vi "line_spectrum.vi"(1 "Image":dbl[][](graph)=array476x2048[974848 elements]) -> (0 "Mean intensity per pixel":cluster{"Ramp Pattern":dbl[], dbl[]}[](graph)=[{"Ramp Pattern"=array[2048 elements], array[2048 elements]}, {"Ramp Pattern"=[767.5, 767.5], [0.0, 100.0]}, {"Ramp Pattern"=[932.5, 932.5], [0.0, 100.0]}, {"Ramp Pattern"=[850.0, 850.0], [0.0, 100.0]}])   [LabVIEW 2017]
uses:
  <vilib>/Analysis/1siggen.llb/Ramp Pattern by Samples.vi
  <vilib>/Analysis/baseanly.llb/Mean (DBL).vi
  <vilib>/Analysis/NI_AALBase.lvlib
panel:
  out "MaxPI (%)":dbl=87.1199407497374 format="%0.1f"
  in  "Source Bandwidth (nm)":i32=165
  in  "Source Center wavelength (nm)":i32=850
  in  "Spec. Bandwidth (nm)":i32=180
  in  "Spec. Center wavelength (nm)":i32=840
  out "MPI (%)":dbl=43.9106688028624 format="%0.1f"
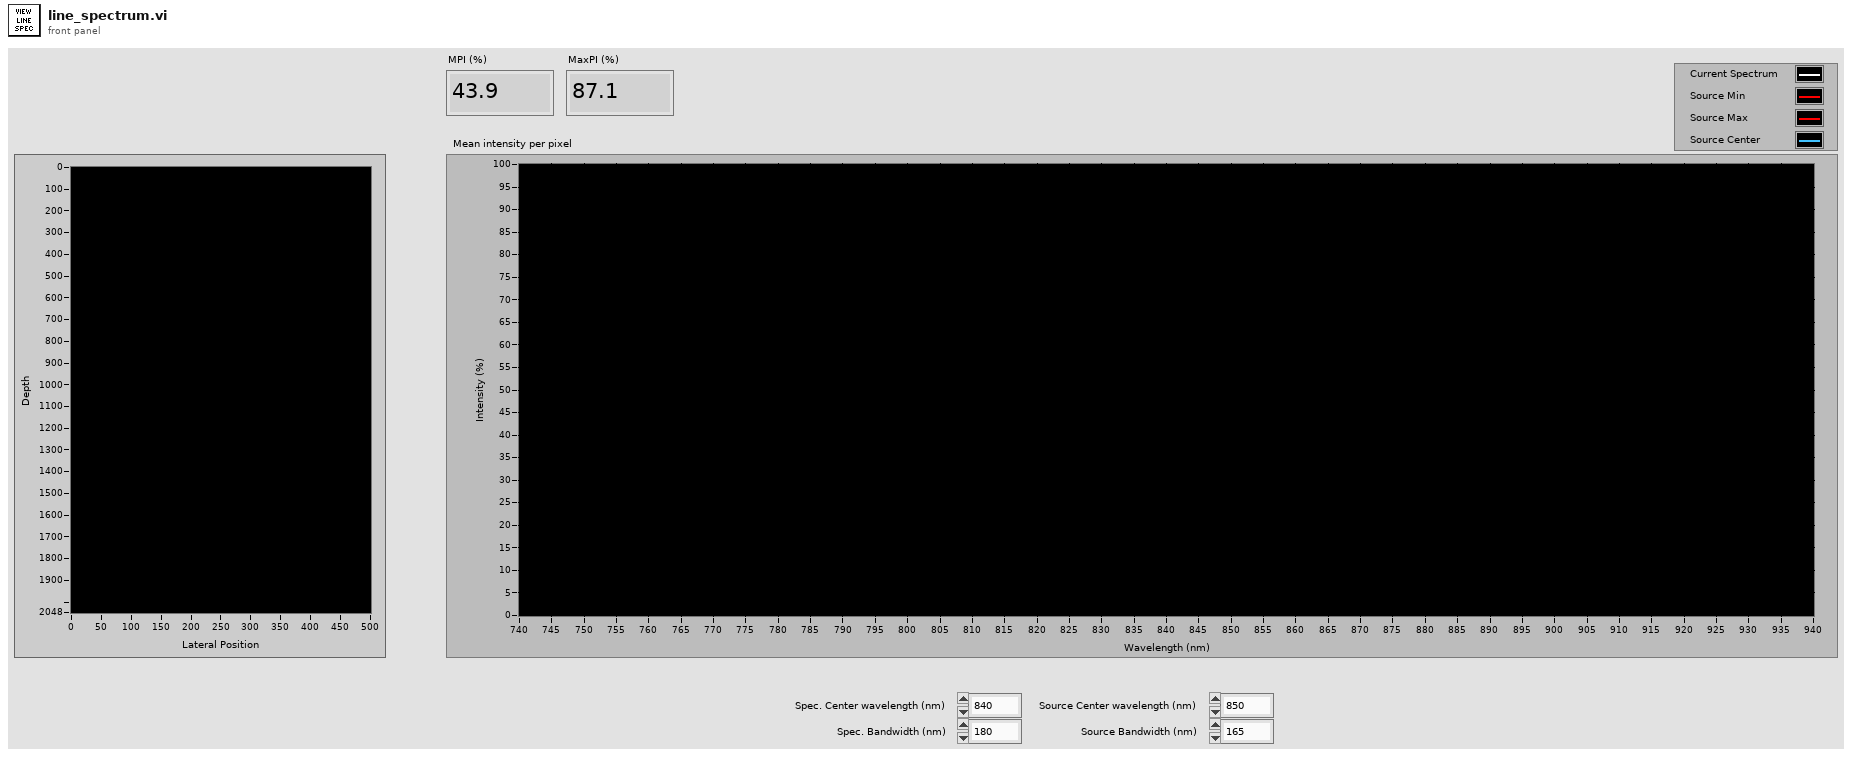
[diagram p1: front panel]
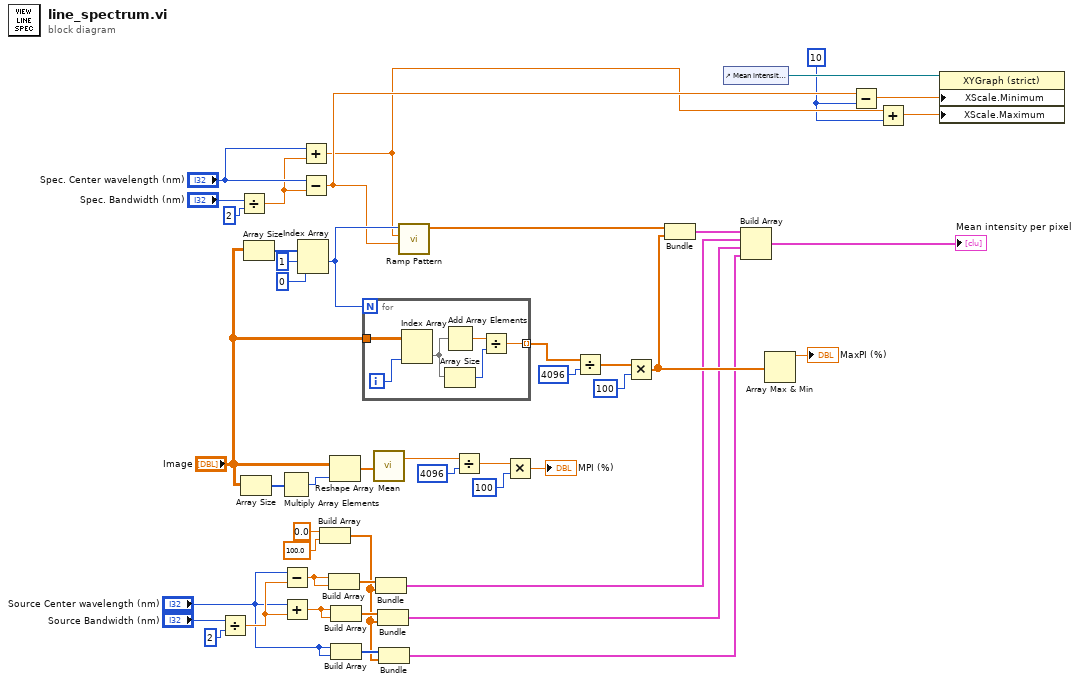
[diagram p0: block diagram]
diagram:
  w1 = 10
  n1 = Divide(x="Source Bandwidth (nm)", y=2) -> (x/y=w24:dbl)
  n2 = Divide(x="Spec. Bandwidth (nm)", y=2) -> (x/y=w26:dbl)
  n3 = Array Size(array="Image") -> (size(s)=w46:i32[])
  n4 = Array Size(array="Image") -> (size(s)=w43:i32[])
  n5 = Multiply Array Elements(1:w46) -> (0:w45:i32)
  n6 = Subtract(x="Source Center wavelength (nm)", y=w24) -> (x-y=w20:dbl)
  n7 = Add(x="Source Center wavelength (nm)", y=w24) -> (x+y=w17:dbl)
  n8 = Index Array(array=w43, index #1=1 ("index"), index #2=0 ("index")) -> (element #1=w39:i32)  [unwired: 1 out]
  n9 = Add(x="Spec. Center wavelength (nm)", y=w26) -> (x+y=w2:dbl)
  n10 = Subtract(x="Spec. Center wavelength (nm)", y=w26) -> (x-y=w3:dbl)
  n11 = Build Array(0.0 ("element"), 100.0 ("element")) -> (w10:dbl[])
  n12 = Build Array(w20, w20) -> (w16:dbl[])
  n13 = Reshape Array("Image", w45) -> (w8:dbl[])
  n14 = Build Array(w17, w17) -> (w15:dbl[])
  n15 = Build Array("Source Center wavelength (nm)", "Source Center wavelength (nm)") -> (w11:i32[])
  n16 = for {
    N: w39 -> [_]
    tunnel: "Image" -> [w53]
    tunnel: [w51] -> w38 mode=indexing
    i -> [w50]
    n17 = Index Array(array=w53, index (col)=w50) -> (element=w49:dbl[])  [unwired: 1 in]
    n18 = Add Array Elements(numeric array=w49) -> (sum=w52:dbl)
    n19 = Array Size(array=w49) -> (size(s)=w48:i32)
    n20 = Divide(x=w52, y=w48) -> (x/y=w51:dbl)
  }
  n21 = call-poly <vilib>:"Mean.vi"("X"=w8) -> ("mean"=w31:dbl)  [unwired: 1 out]
  n22 = Bundle(w16, w10) -> (w14:cluster{dbl[], dbl[]})  [unwired: 1 in]
  n23 = Bundle(w15, w10) -> (w13:cluster{dbl[], dbl[]})  [unwired: 1 in]
  n24 = Bundle(w11, w10) -> (w9:cluster{i32[], dbl[]})  [unwired: 1 in]
  n25 = call-poly <vilib>:"Ramp Pattern.vi"("start"=w3, "end"=w2, "samples"=w39) -> ("Ramp Pattern"=w41:dbl[])  [unwired: 7 in, 1 out]
  n26 = Divide(x=w31, y=4096) -> (x/y=w33:dbl)
  n27 = Multiply(x=w33, y=100) -> (x*y=→"MPI (%)":dbl)
  n28 = Divide(x=w38, y=4096) -> (x/y=w36:dbl[])
  n29 = Multiply(x=w36, y=100) -> (x*y=w47:dbl[])
  n30 = Bundle("Ramp Pattern"=w41, w47) -> (w22:cluster{"Ramp Pattern":dbl[], dbl[]})  [unwired: 1 in]
  n31 = control-ref of="Mean intensity per pixel"() -> (w6:refnum<vi>)
  n32 = Build Array(w22, w14, w13, w9) -> (→"Mean intensity per pixel":cluster{"Ramp Pattern":dbl[], dbl[]}[])
  n33 = Array Max & Min(array=w47) -> (max value=→"MaxPI (%)":dbl)  [unwired: 3 out]
  n34 = Subtract(x=w3, y=w1) -> (x-y=w5:dbl)
  n35 = Add(x=w2, y=w1) -> (x+y=w4:dbl)
  n36 = property class="XYGraph (strict)"(reference=w6, "XScale.Minimum"=w5, "XScale.Maximum"=w4) -> ()  [unwired: 1 in, 2 out]
